vi "SPC_restart_measurement.vi"(8 "Error In":errorcluster, 10 "Module No":i16 min=0 max=7 step=1, 11 "DLL Path":path) -> (0 "Error Out":errorcluster, 2 "Module No":i16 min=0 max=7 step=1, 3 "DLL Path":path)   [LabVIEW 2023]
doc: "The procedure is used to restart a measurement that was paused by SPC_pause_measurement on the SPC module ‘mod_no’.\nBecause of hardware differences the procedure's action varies for different SPC module types.\nFor all SPC module types (except SPC-6x0/13x/830/140/930/15x/160 in FIFO modes):\nWhen the sequencer is not enabled (normal measurement):\n - the repeat and collection timers are started,\n - the SPC is armed (photon collection is started).\nWhen the sequencer is enabled:\n -an error is returned, this measurement can’t be restarted\nFor SPC-6x0/13x/830/140/930/15x/160 in FIFO mode:\n The procedure should not be used for FIFO modules.\n\ninfo@becker-hickl.com"
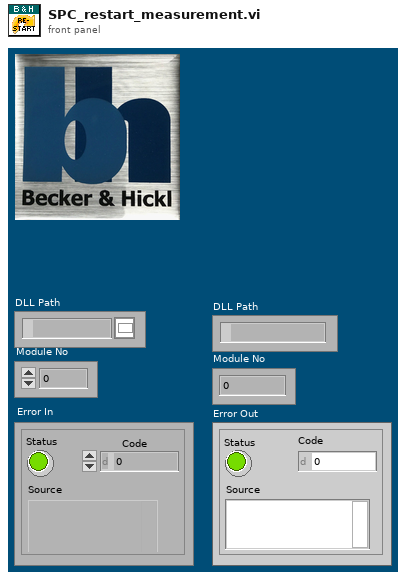
[diagram p1: front panel]
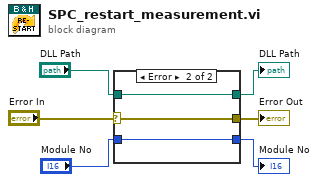
[diagram p0: block diagram]
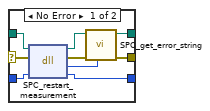
[diagram p2: hidden frame]
diagram:
  n1 = case shown="Error" "Error In" {
    selector: "Error In" -> [w13 w17]
    tunnel: [w9 w17] -> w6
    tunnel: [w12 w18] -> w5
    tunnel: "DLL Path" -> [w14 w18]
    tunnel: [w8 w16] -> w2
    tunnel: "Module No" -> [w7 w16]
    frame No Error {
      n2 = dll-call lib="D:/spcm/lib/lab_view/lv10.0/spcm32.dll" fn="SPC_restart_measurement"(path in=w14, error in=w13, "mod_no"=w7) -> (path out=w15:path, error out=w11:errorcluster, "return type"=w10:i16, "mod_no"=w8:i16)  [unwired: 1 in]
      n3 = call "SPC_get_error_string.vi"("ErrorID"=w10, "Error In"=w11, "DLL Path"=w15) -> ("Error Out"=w9:errorcluster, "DLL Path"=w12:path)  [unwired: 6 in, 1 out]
    }
    frame Error {
    }
  }
  "DLL Path" <- w5
  "Error Out" <- w6
  "Module No" <- w2
